vi "Create SSC.vi"(6 "sample rate":dbl=1000.0 format="%#_6p", 7 "OVS":u8=16, 8 "error in (no error)":errorcluster) -> (0 "error out":errorcluster, 3 "Digital Waveform Graph":digitalwaveform(graph))   [LabVIEW 2013]
uses:
  <vilib>/Waveform/DWDTOps.llb/Digital Pattern Generator (Single Value).vi
  <vilib>/Waveform/DWDTOps.llb/DWDT Append Digital Samples.vi
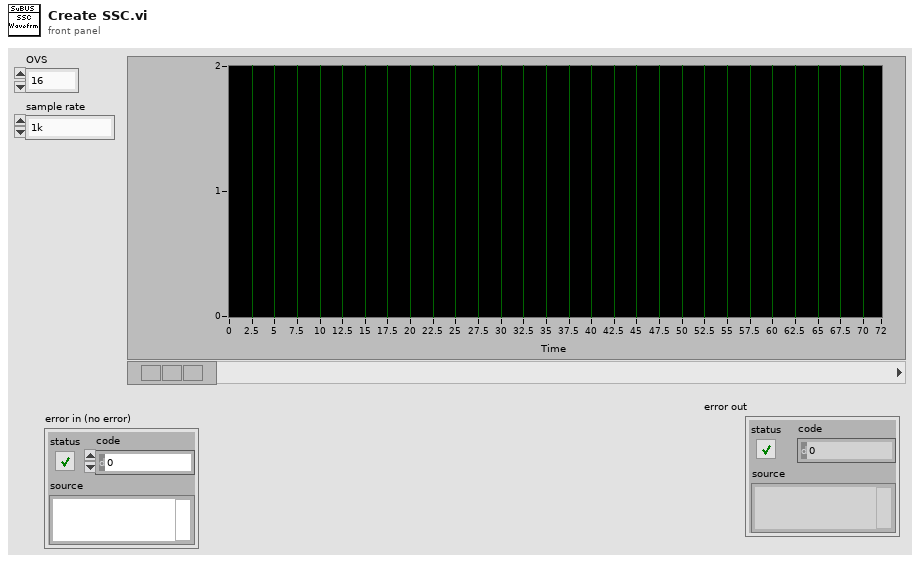
[diagram p1: front panel]
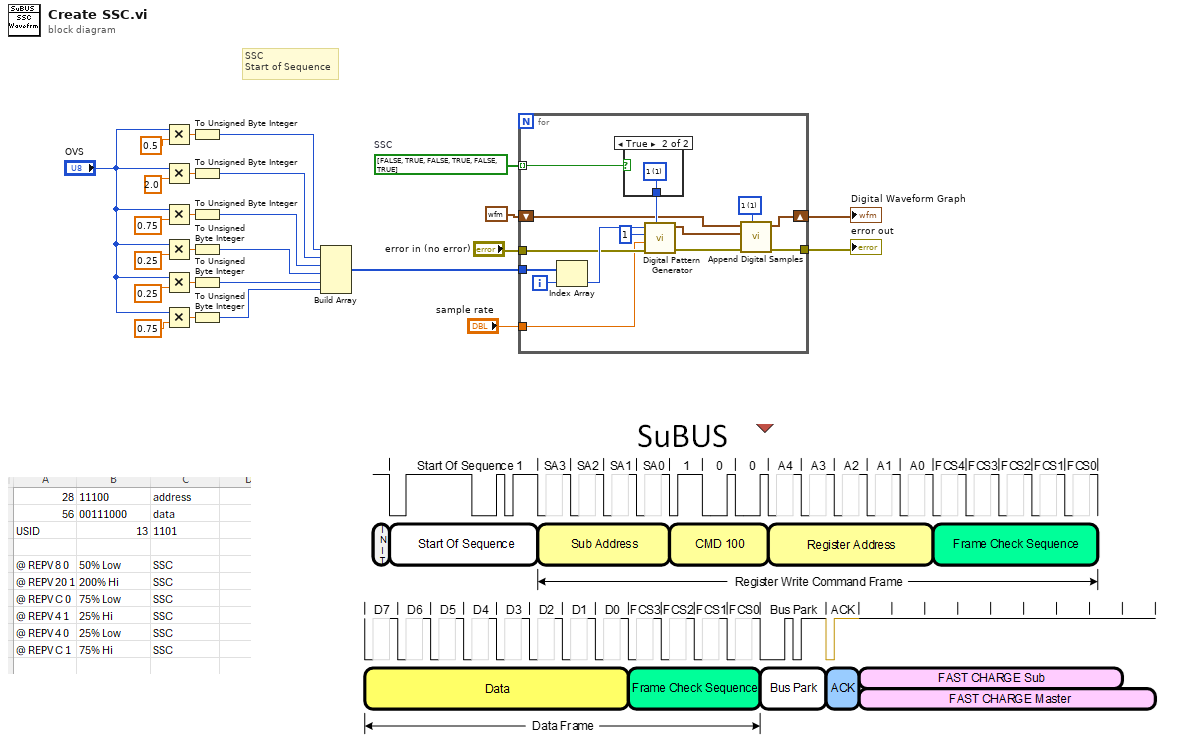
[diagram p0: block diagram]
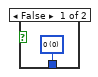
[diagram p2: hidden frame]
diagram:
  w1 = bool[] [FALSE, TRUE, FALSE, TRUE, FALSE, TRUE]  # SSC
  # "SSC\nStart of Sequence"
  n1 = Multiply(x="OVS", y=0.5) -> (x*y=w26:dbl)
  n2 = Multiply(x="OVS", y=2.0) -> (x*y=w24:dbl)
  n3 = Multiply(x="OVS", y=0.75) -> (x*y=w22:dbl)
  n4 = Multiply(x="OVS", y=0.25) -> (x*y=w20:dbl)
  n5 = Multiply(x="OVS", y=0.25) -> (x*y=w18:dbl)
  n6 = Multiply(x="OVS", y=0.75) -> (x*y=w16:dbl)
  n7 = To Unsigned Byte Integer(number=w26) -> (unsigned 8bit integer=w14:u8)
  n8 = To Unsigned Byte Integer(number=w24) -> (unsigned 8bit integer=w13:u8)
  n9 = To Unsigned Byte Integer(number=w22) -> (unsigned 8bit integer=w12:u8)
  n10 = To Unsigned Byte Integer(number=w20) -> (unsigned 8bit integer=w11:u8)
  n11 = To Unsigned Byte Integer(number=w18) -> (unsigned 8bit integer=w10:u8)
  n12 = To Unsigned Byte Integer(number=w16) -> (unsigned 8bit integer=w9:u8)
  n13 = Build Array(w14, w13, w12, w11, w10, w9) -> (w8:u8[])
  n14 = for {
    tunnel: w8 -> [w40]
    tunnel: w1 -> [w37] mode=indexing
    shift-right: [w31] -> w3
    shift-left: digitalwaveform {"t0"=timestamp(0 s since 1904-01-01), "dt"=0.0, "Y"={"transitions"=[], "data"=[]}} ("digital waveform out") -> [w30]
    tunnel: "error in (no error)" -> [w29]
    tunnel: [w28] -> w4
    tunnel: "sample rate" -> [w27]
    i -> [w39]
    w34 = u8 1 items=["0", "1", "Z", "L", "H", "X", "T", "V"] ("default value")
    n15 = Index Array(array=w40, index=w39) -> (element=w35:u8)
    n16 = case shown="True" w37 {
      tunnel: [w41 w42] -> w36
      frame False {
        w41 = u8 0 items=["0", "1", "Z", "L", "H", "X", "T", "V"] ("value")
      }
      frame True {
        w42 = u8 1 items=["0", "1", "Z", "L", "H", "X", "T", "V"] ("value")
      }
    }
    n17 = call-poly <vilib>:"Digital Pattern Generator.vi"("value"=w36, "error in (no error)"=w29, "sample rate"=w27, "number of signals"=u32 1, "number of samples"=w35) -> ("error out"=w33:errorcluster, "digital waveform"=w32:digitalwaveform)  [unwired: 5 in]
    n18 = call-poly <vilib>:"Append Digital Samples.vi"("default value"=w34, "error in (no error)"=w33, "digital waveform B"=w32, "digital waveform A"=w30) -> ("error out"=w28:errorcluster, "digital waveform out"=w31:digitalwaveform)  [unwired: 6 in]
  }
  "error out" <- w4
  "Digital Waveform Graph" <- w3
